vi "Error Message.vi"(0 "VISA resource name":refnum<visa-resource-name>, 11 "error in (no error)":errorcluster {"code" format="%.0x"}) -> (4 "VISA resource name out":refnum<visa-resource-name>, 15 "error out":errorcluster {"code" format="%.0x"})   [LabVIEW 2015, in "Voltech PM1000+.lvlib"]
doc: "This VI contains all the intrument specific error codes and descriptions. Use this VI after executing several instrument driver VIs to recognize and display any errors that may have occurred."
uses:
  <instrlib>/Voltech PM1000+/Voltech PM1000+.lvlib
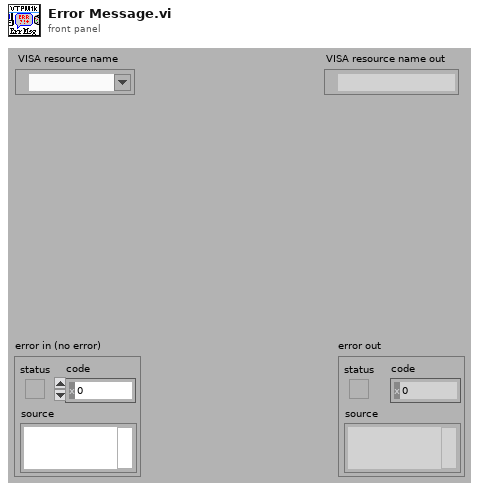
[diagram p1: front panel]
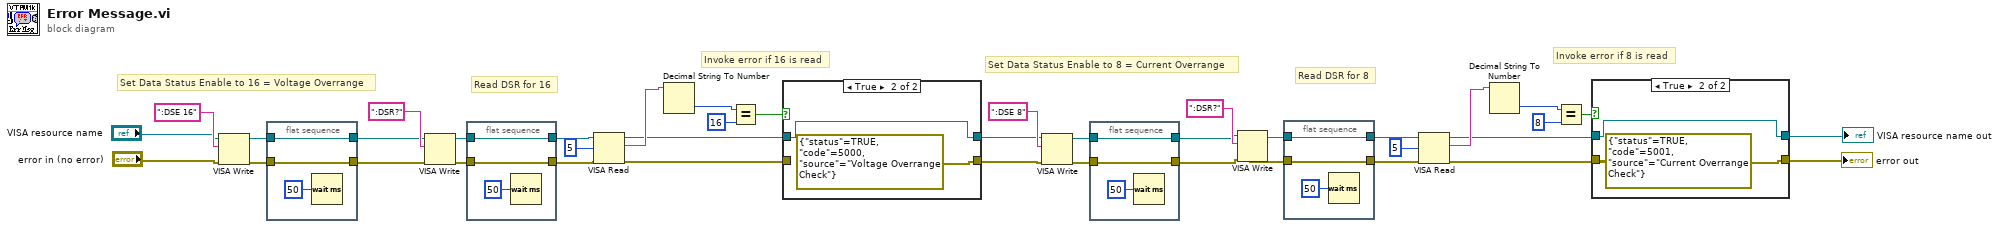
[diagram p0: block diagram]
diagram:
  # "Invoke error if 8 is read"
  # "Read DSR for 8"
  # "Set Data Status Enable to 8 = Current Overrange"
  # "Invoke error if 16 is read"
  # "Read DSR for 16"
  # "Set Data Status Enable to 16 = Voltage Overrange"
  n1 = VISA Write(VISA resource name="VISA resource name", write buffer=":DSE 16", error in (no error)="error in (no error)") -> (VISA resource name out=w12:refnum<visa-resource-name>, error out=w11:errorcluster)  [unwired: 1 out]
  n2 = flat-sequence {
    tunnel: [w43] -> w10
    tunnel: w12 -> [w43]
    tunnel: [w42] -> w9
    tunnel: w11 -> [w42]
    frame #0 {
      n3 = Wait (ms)(milliseconds to wait=50) -> ()  [unwired: 1 out]
    }
  }
  n4 = VISA Write(VISA resource name=w10, write buffer=":DSR?", error in (no error)=w9) -> (VISA resource name out=w16:refnum<visa-resource-name>, error out=w14:errorcluster)  [unwired: 1 out]
  n5 = flat-sequence {
    tunnel: [w46] -> w15
    tunnel: w16 -> [w46]
    tunnel: [w45] -> w13
    tunnel: w14 -> [w45]
    frame #0 {
      n6 = Wait (ms)(milliseconds to wait=50) -> ()  [unwired: 1 out]
    }
  }
  n7 = VISA Read(VISA resource name=w15, byte count=5, error in (no error)=w13) -> (VISA resource name out=w30:refnum<visa-resource-name>, read buffer=w35:string, error out=w32:errorcluster)  [unwired: 1 out]
  n8 = Decimal String To Number(string=w35) -> (number=w34:i32)  [unwired: 2 in, 1 out]
  n9 = Equal?(x=w34, y=16) -> (x = y?=w31:bool)
  n10 = case shown="True" w31 {
    tunnel: w32 -> [w48 _]
    tunnel: [w48 errorcluster {"status"=TRUE, "code"=5000, "source"="Voltage Overrange Check"} ("error out")] -> w22
    tunnel: w30 -> [w47 w49]
    tunnel: [w47 w49] -> w23
    frame False {
    }
    frame True {
    }
  }
  n11 = VISA Write(VISA resource name=w23, write buffer=":DSE 8", error in (no error)=w22) -> (VISA resource name out=w4:refnum<visa-resource-name>, error out=w2:errorcluster)  [unwired: 1 out]
  n12 = flat-sequence {
    tunnel: [w53] -> w3
    tunnel: w4 -> [w53]
    tunnel: [w52] -> w1
    tunnel: w2 -> [w52]
    frame #0 {
      n13 = Wait (ms)(milliseconds to wait=50) -> ()  [unwired: 1 out]
    }
  }
  n14 = VISA Write(VISA resource name=w3, write buffer=":DSR?", error in (no error)=w1) -> (VISA resource name out=w5:refnum<visa-resource-name>, error out=w7:errorcluster)  [unwired: 1 out]
  n15 = flat-sequence {
    tunnel: [w54] -> w8
    tunnel: [w56] -> w6
    tunnel: w7 -> [w56]
    tunnel: w5 -> [w54]
    frame #0 {
      n16 = Wait (ms)(milliseconds to wait=50) -> ()  [unwired: 1 out]
    }
  }
  n17 = VISA Read(VISA resource name=w8, byte count=5, error in (no error)=w6) -> (VISA resource name out=w21:refnum<visa-resource-name>, read buffer=w26:string, error out=w20:errorcluster)  [unwired: 1 out]
  n18 = Decimal String To Number(string=w26) -> (number=w25:i32)  [unwired: 2 in, 1 out]
  n19 = Equal?(x=w25, y=8) -> (x = y?=w17:bool)
  n20 = case shown="True" w17 {
    tunnel: w20 -> [w58 _]
    tunnel: [w58 errorcluster {"status"=TRUE, "code"=5001, "source"="Current Overrange Check"} ("error out")] -> w18
    tunnel: w21 -> [w57 w59]
    tunnel: [w57 w59] -> w19
    frame False {
    }
    frame True {
    }
  }
  "VISA resource name out" <- w19
  "error out" <- w18
